vi "Send Message.vi"(8 "error in (no error)":errorcluster caption="错误输入（无错误）", 11 "Bark 输入":refnum<class "Bark.lvclass">) -> (0 "error out":errorcluster caption="错误输出", 3 "Bark 输出":refnum<class "Bark.lvclass">)   [LabVIEW 2016, in "Bark.lvlib" / "Bark.lvclass"]
uses:
  Bark.lvclass
  Bark.lvclass/Bark.ctl
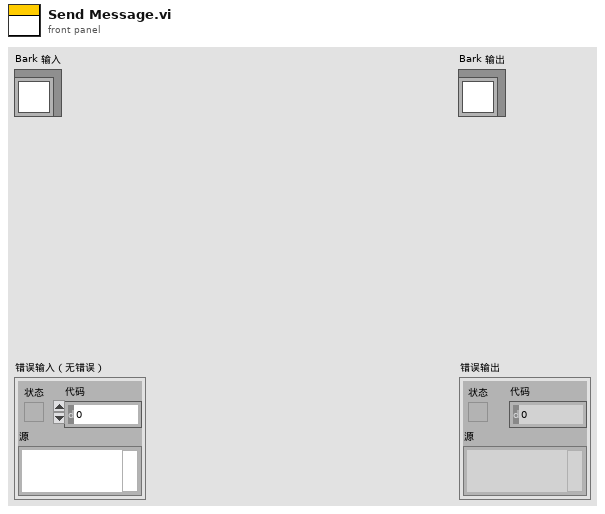
[diagram p1: front panel]
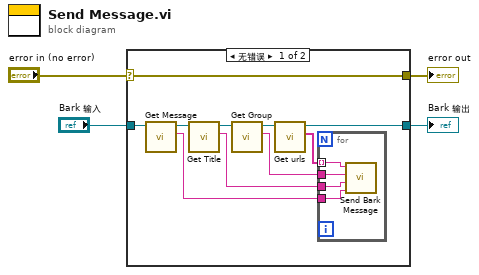
[diagram p0: block diagram]
diagram:
  n1 = case shown="无错误" "error in (no error)" {
    selector: "error in (no error)" -> [w14 w20]
    tunnel: [w14 w20] -> w3
    tunnel: [w13 w19] -> w1
    tunnel: "Bark 输入" -> [w6 w19]
    frame No Error {
      n2 = call "Get Message.vi"("Bark in"=w6) -> ("Message"=w10:string, "Bark out"=w7:refnum<class "Bark.lvclass">)  [unwired: 9 in]
      n3 = call "Get Title.vi"("Bark in"=w7) -> ("Title"=w11:string, "Bark out"=w8:refnum<class "Bark.lvclass">)  [unwired: 9 in]
      n4 = call "Get Group.vi"("Bark in"=w8) -> ("Group"=w9:string, "Bark out"=w5:refnum<class "Bark.lvclass">)  [unwired: 9 in]
      n5 = call "Get urls.vi"("Bark in"=w5) -> ("urls"=w12:string[], "Bark out"=w13:refnum<class "Bark.lvclass">)  [unwired: 9 in]
      n6 = for {
        tunnel: w12 -> [w18] mode=indexing
        tunnel: w11 -> [w17]
        tunnel: w10 -> [w16]
        tunnel: w9 -> [w15]
        n7 = call "Send Bark Message.vi"("Message"=w16, "Title"=w17, "Group"=w15, "Url"=w18) -> ()  [unwired: 8 in]
      }
    }
    frame Error {
    }
  }
  "error out" <- w3
  "Bark 输出" <- w1
